vi "New Results.vi"(6 "Parameters":refnum<class "Analyze Parameter Base.lvclass">[](array[class]), 8 "error in (no error)":errorcluster, 9 "Image Nr.":i32, 10 "Results":refnum<class "Analyze Results Base.lvclass">[](array[class]), 11 "HIJ Vision Display in":refnum<class "HIJ Vision Display.lvclass">) -> (0 "error out":errorcluster, 3 "HIJ Vision Display out":refnum<class "HIJ Vision Display.lvclass">)   [LabVIEW 2014, in "HIJ Vision Display.lvlib" / "HIJ Vision Display.lvclass"]
uses:
  HIJ Vision Display.lvclass
  Results and Overlays/Results Base/Analyze Results Base.lvclass
  Analyze Parameter/Analyze Parameter Base/Analyze Parameter Base.lvclass
  HIJ Vision Display.lvclass/HIJ Vision Display.ctl
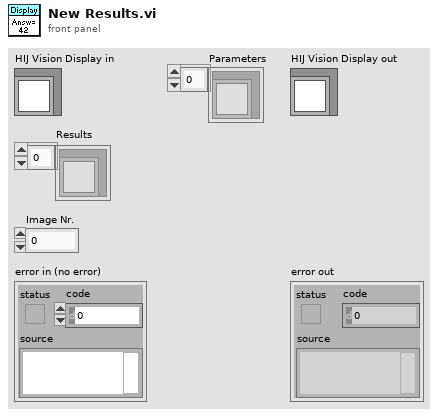
[diagram p1: front panel]
types:
  T1 = typedef "IMAQ Image.ctl" = refnum<image>
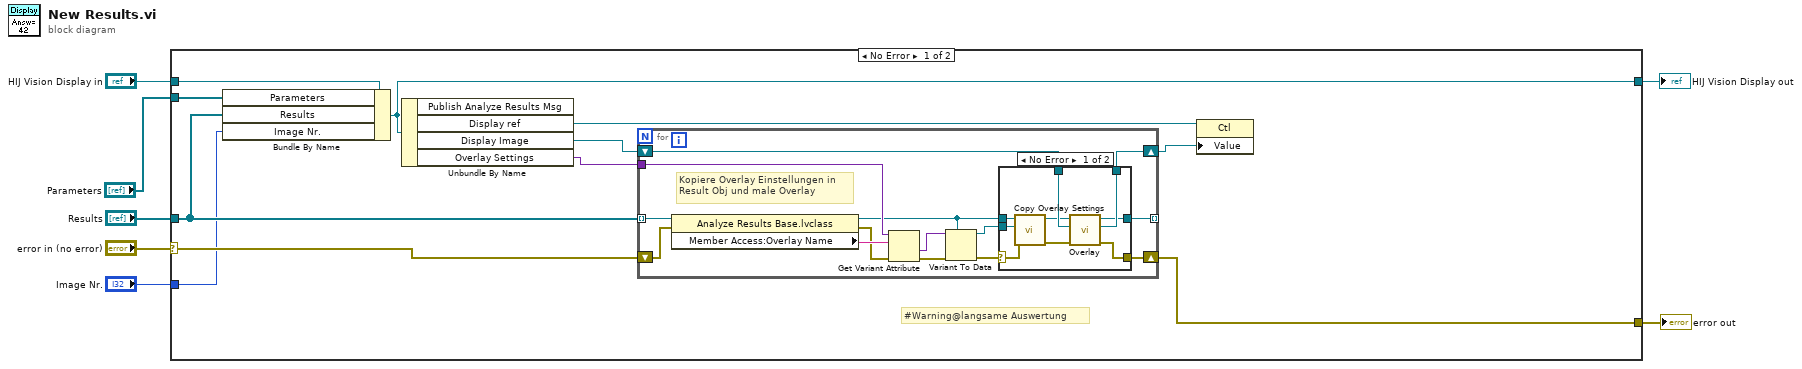
[diagram p0: block diagram]
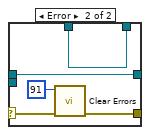
[diagram p2: hidden frame]
diagram:
  n1 = case shown="No Error" "error in (no error)" {
    selector: "error in (no error)" -> [w16 w48]
    tunnel: [w15 w48] -> w6
    tunnel: [w11 w47] -> w4
    tunnel: "HIJ Vision Display in" -> [w18 w47]
    tunnel: "Results" -> [w9 _]
    tunnel: "Image Nr." -> [w8 _]
    tunnel: "Parameters" -> [w10 _]
    frame No Error {
      # "#Warning@langsame Auswertung"
      n2 = Bundle By Name(cluster=w18, "Parameters"=w10, "Results"=w9, "Image Nr."=w8) -> (w11:refnum<class "HIJ Vision Display.lvclass">)
      n3 = Unbundle By Name(w11) -> ("Display ref"=w14:refnum<vi>, "Display Image"=w17:T1, "Overlay Settings"=w12:variant)  [unwired: 1 out]
      n4 = for {
        shift-right: [w30] -> w13
        shift-left: w17 -> [w31]
        tunnel: w9 -> [w32] mode=indexing
        tunnel: [w29] -> _ mode=indexing
        shift-right: [w28] -> w15
        shift-left: w16 -> [w25]
        tunnel: w12 -> [w27]
        # "Kopiere Overlay Einstellungen in \nResult Obj und male Overlay"
        n5 = property class="Analyze Results Base.lvclass"(reference=w32, error in=w25) -> (reference out=w22:refnum<class "Analyze Results Base.lvclass">, error out=w23:errorcluster, "Member Access:Overlay Name"=w26:string)
        n6 = Get Variant Attribute(Variant=w27, name=w26, error in=w23) -> (value=w19:variant, error out=w24:errorcluster)  [unwired: 1 in, 2 out]
        n7 = Variant To Data(error in=w24, type=w22, Variant=w19) -> (data=w21:refnum<class "Analyze Results Base.lvclass">, error out=w20:errorcluster)
        n8 = case shown="No Error" w20 {
          selector: w20 -> [w33 w44]
          tunnel: w31 -> [w41 w45]
          tunnel: [w40 w45] -> w30
          tunnel: [w39 w46] -> w29
          tunnel: [w38 w43] -> w28
          tunnel: w22 -> [w37 w46]
          tunnel: w21 -> [w35 _]
          frame No Error {
            n9 = call "Copy Overlay Settings.vi"("error in (no error)"=w33, "Source"=w35, "Destination"=w37) -> ("error out"=w34:errorcluster, "Analyze Results Base out"=w36:refnum<class "Analyze Results Base.lvclass">)  [unwired: 7 in]
            n10 = call-dynamic "Overlay.vi"("error in (no error)"=w34, "Image In"=w41, "Overlay Base in"=w36) -> ("error out"=w38:errorcluster, "Image out"=w40:T1, "Overlay Base out"=w39:refnum<class "Analyze Results Base.lvclass">)  [unwired: 6 in]
          }
          frame Error {
            n11 = call <vilib>:"Clear Errors.vi"("error in (no error)"=w44, "specific error code to clear (0: all)"=91) -> ("error out"=w43:errorcluster)  [unwired: 4 in, 1 out]
          }
        }
      }
      n12 = property class="Ctl"(reference=w14, "Value"=w13) -> ()  [unwired: 1 in, 2 out]
    }
    frame Error {
    }
  }
  "error out" <- w6
  "HIJ Vision Display out" <- w4
